vi "gpsdata.vi"() -> (3 "GPS DATA 2":T1={"type"="None", "x_lcc"=-59.06772232055664, "y_lcc"=-26.082616806030273, "latdev"=0.0, "londev"=0.0, "sats"=0, "gps_l1_ranges"=0, "gps_l1_mask_ranges"=0, "gps_l2_mask_ranges"=0, "Heading"=89.78975677490234, "lon"=0.0, "lat"=0.0, "time"="None", "hgps"=89.78975677490234, "lag"=89.78975677490234, "MAP"="None"} {"lag" format="%#_5g"; "hgps" format="%#_5g"; "lat" format="%#_11g"; "lon" format="%#_11g"; "Heading" format="%#_5g"; "latdev" format="%#_4g"; "londev" format="%#_4g"})   [LabVIEW 2015]
uses:
  G_ALL.vi
  G_LCM.vi
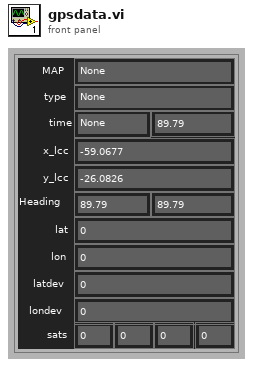
[diagram p1: front panel]
types:
  T1 = cluster{"type":string, "x_lcc":dbl, "y_lcc":dbl, "latdev":sgl, "londev":sgl, "sats":u8, "gps_l1_ranges":u8, "gps_l1_mask_ranges":u8, "gps_l2_mask_ranges":u8, "Heading":dbl, "lon":sgl, "lat":sgl, "time":string, "hgps":dbl, "lag":dbl, "MAP":string}
  T2 = cluster{"hash":i64, "sys time":i64, "time":dbl, "x":dbl, "y":dbl, "h":dbl, "numSV":i32, "postype":i32, "lag":i32, "hordev":dbl, "lat":dbl, "lon":dbl, "hgt":dbl, "map_idx":i32}
  T3 = cluster{"Steer_input":dbl, "Steer_output":dbl, "VS_des":dbl, "VS_can":dbl, "heading":dbl, "auto":bool, "run":bool, "x":dbl, "y":dbl}
  T4 = cluster{"hash":i64, "sys time":i64, "time":dbl, "speed":dbl, "heading":dbl, "lat":dbl, "lon":dbl}
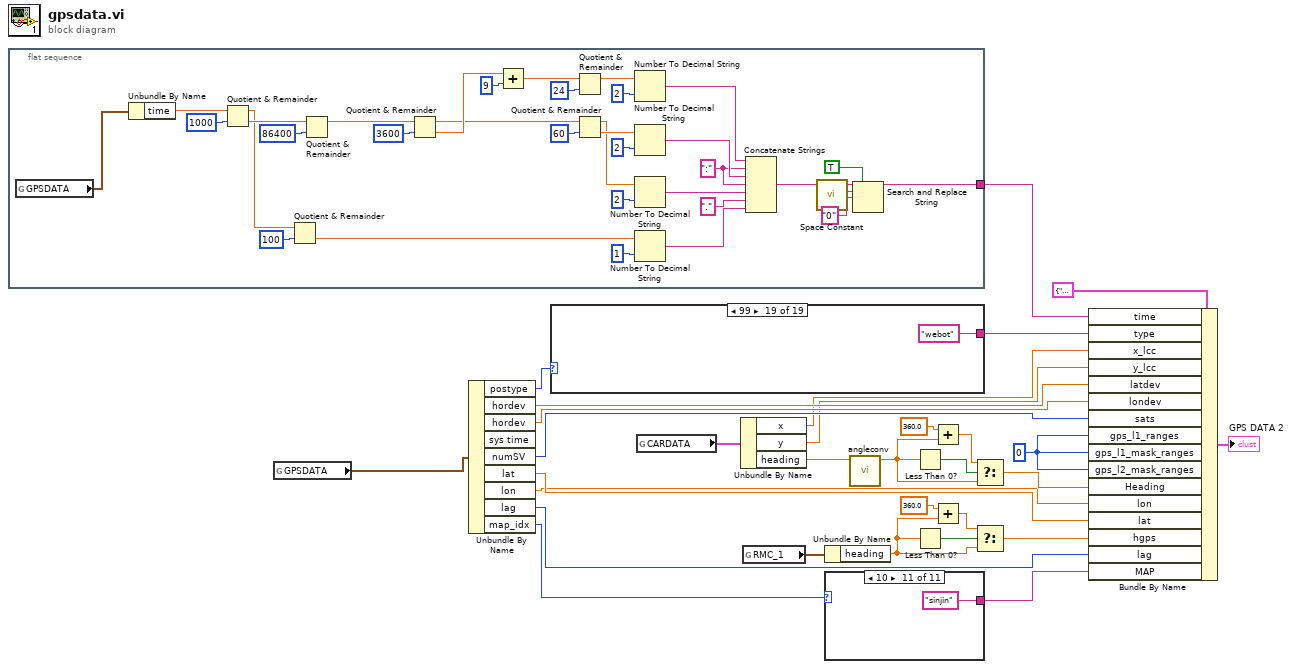
[diagram p0: block diagram]
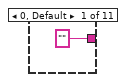
[diagram p2: hidden frame]
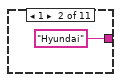
[diagram p3: hidden frame]
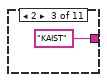
[diagram p4: hidden frame]
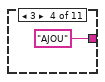
[diagram p5: hidden frame]
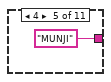
[diagram p6: hidden frame]
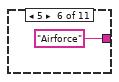
[diagram p7: hidden frame]
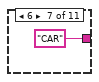
[diagram p8: hidden frame]
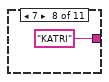
[diagram p9: hidden frame]
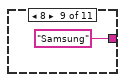
[diagram p10: hidden frame]
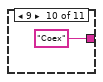
[diagram p11: hidden frame]
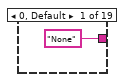
[diagram p12: hidden frame]
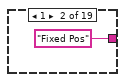
[diagram p13: hidden frame]
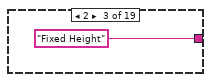
[diagram p14: hidden frame]
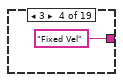
[diagram p15: hidden frame]
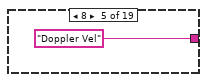
[diagram p16: hidden frame]
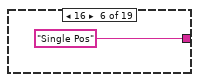
[diagram p17: hidden frame]
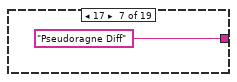
[diagram p18: hidden frame]
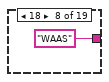
[diagram p19: hidden frame]
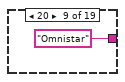
[diagram p20: hidden frame]
diagram:
  w11 = u8 0 ("gps_l2_mask_ranges")
  n1 = flat-sequence {
    tunnel: [w36] -> w6
    frame #0 {
      w51 = ":" ("string")
      n2 = global read "G_ALL.vi" "GPSDATA"() -> (w31:T2)
      n3 = Unbundle By Name(w31) -> ("time"=w32:dbl)
      n4 = Quotient & Remainder(x=w32, y=u32 1000) -> (x-y*floor(x/y)=w39:dbl, floor(x/y)=w44:dbl)
      n5 = Quotient & Remainder(x=w39, y=u32 100) -> (floor(x/y)=w38:dbl)  [unwired: 1 out]
      n6 = Quotient & Remainder(x=w44, y=u32 86400) -> (x-y*floor(x/y)=w48:dbl)  [unwired: 1 out]
      n7 = Quotient & Remainder(x=w48, y=u32 3600) -> (x-y*floor(x/y)=w47:dbl, floor(x/y)=w63:dbl)
      n8 = Add(x=w63, y=u32 9) -> (x+y=w61:dbl)
      n9 = Quotient & Remainder(x=w61, y=u32 24) -> (x-y*floor(x/y)=w58:dbl)  [unwired: 1 out]
      n10 = Quotient & Remainder(x=w47, y=u32 60) -> (x-y*floor(x/y)=w46:dbl, floor(x/y)=w56:dbl)
      n11 = Number To Decimal String(number=w58, width (-)=i16 2) -> (decimal integer string=w53:string)
      n12 = Number To Decimal String(number=w56, width (-)=i16 2) -> (decimal integer string=w52:string)
      n13 = Number To Decimal String(number=w46, width (-)=i16 2) -> (decimal integer string=w50:string)
      n14 = Number To Decimal String(number=w38, width (-)=i16 1) -> (decimal integer string=w42:string)
      n15 = Concatenate Strings(w53, w51, w52, w51, w50, "." ("string"), w42) -> (w37:string)
      n16 = call <vilib>:"Space Constant.vi"() -> ("String"=w35:string)
      n17 = Search and Replace String(replace all?=TRUE ("replace all? (F)"), input string=w37, search string=w35, replace string="0" ("replace string (\"\")")) -> (result string=w36:string)  [unwired: 4 in, 3 out]
    }
  }
  n18 = global read "G_ALL.vi" "GPSDATA"() -> (w1:T2)
  n19 = Unbundle By Name(w1) -> ("postype"=w30:i32, "hordev"=w29:dbl, "hordev"=w28:dbl, "numSV"=w27:i32, "lat"=w10:dbl, "lon"=w9:dbl, "lag"=w8:i32, "map_idx"=w2:i32)  [unwired: 1 out]
  n20 = case shown="99" w30 {
    tunnel: ["None" "Fixed Pos" "Fixed Height" "Fixed Vel" "Doppler Vel" "Single Pos" "Pseudoragne Diff" "WAAS" "Omnistar" "Floating L1 Ambiguity" "Floating Iono-free" "Floating Narrow-lane Amb" "Integer L1 Ambiguity" "Integer Wide-lane Amb" "Integer Narrow-lane Amb" "RTK Direct-init by INS" "INS levarm compensated" "OmniSTAR HP position" "webot"] -> w7
    frame 0, Default {
    }
    frame 1 {
    }
    frame 2 {
    }
    frame 3 {
    }
    frame 8 {
    }
    frame 16 {
    }
    frame 17 {
    }
    frame 18 {
    }
    frame 20 {
    }
    frame 32 {
    }
    frame 33 {
    }
    frame 34 {
    }
    frame 48 {
    }
    frame 49 {
    }
    frame 50 {
    }
    frame 51 {
    }
    frame 52 {
    }
    frame 64 {
    }
    frame 99 {
    }
  }
  n21 = global read "G_ALL.vi" "CARDATA"() -> (w3:T3)
  n22 = Unbundle By Name(w3) -> ("x"=w15:dbl, "y"=w16:dbl, "heading"=w22:dbl)
  n23 = global read "G_LCM.vi" "RMC_1"() -> (w5:T4)
  n24 = Unbundle By Name(w5) -> ("heading"=w4:dbl)
  n25 = case shown="10" w2 {
    tunnel: ["" ("String") "Hyundai" ("String") "KAIST" ("String") "AJOU" ("String") "MUNJI" ("String") "Airforce" ("String") "CAR" ("String") "KATRI" ("String") "Samsung" ("String") "Coex" ("String") "sinjin" ("String")] -> w12
    frame 0, Default {
    }
    frame 1 {
    }
    frame 2 {
    }
    frame 3 {
    }
    frame 4 {
    }
    frame 5 {
    }
    frame 6 {
    }
    frame 7 {
    }
    frame 8 {
    }
    frame 9 {
    }
    frame 10 {
    }
  }
  n26 = call "angleconv.vi"("rad"=w22) -> ("deg"=w23:dbl)  [unwired: 9 in, 1 out]
  n27 = Less Than 0?(x=w23) -> (x < 0?=w25:bool)
  n28 = Less Than 0?(x=w4) -> (x < 0?=w19:bool)
  n29 = Add(x=360.0, y=w23) -> (x+y=w26:dbl)
  n30 = Add(x=360.0, y=w4) -> (x+y=w18:dbl)
  n31 = Select(t=w26, s=w25, f=w23) -> (s? t:f=w21:dbl)
  n32 = Select(t=w18, s=w19, f=w4) -> (s? t:f=w17:dbl)
  n33 = Bundle By Name(cluster=T1 {"type"="None", "x_lcc"=-59.06772232055664, "y_lcc"=-26.082616806030273, "latdev"=0.0, "londev"=0.0, "sats"=0, "gps_l1_ranges"=0, "gps_l1_mask_ranges"=0, "gps_l2_mask_ranges"=0, "Heading"=89.78975677490234, "lon"=0.0, "lat"=0.0, "time"="None", "hgps"=89.78975677490234, "lag"=89.78975677490234, "MAP"="None"} ("GPS DATA 2"), "time"=w6, "type"=w7, "x_lcc"=w15, "y_lcc"=w16, "latdev"=w29, "londev"=w28, "sats"=w27, "gps_l1_ranges"=w11, "gps_l1_mask_ranges"=w11, "gps_l2_mask_ranges"=w11, "Heading"=w21, "lon"=w9, "lat"=w10, "hgps"=w17, "lag"=w8, "MAP"=w12) -> (→"GPS DATA 2":T1)
